vi "EneryPixelInitSingle.vi"(8 "error in (no error)":errorcluster, 11 "MagSpecCamera in":refnum<class "MagSpecCamera.lvclass">) -> (0 "error out":errorcluster, 3 "MagSpecCamera in":refnum<class "MagSpecCamera.lvclass">)   [LabVIEW 2013, in "MagSpecCamera.lvclass"]
uses:
  MagSpecCamera.lvclass
  MagSpecCamera.lvclass/MagSpecCamera.ctl
panel:
  out "Charge Compensation 2":dbl[](graph)
  out "energy dep":dbl[](graph)
  out "Bending angle":dbl[](graph)
  out "Charge Compensation":dbl[](graph)
  out "Momentum [MeV/C]":dbl[](graph)
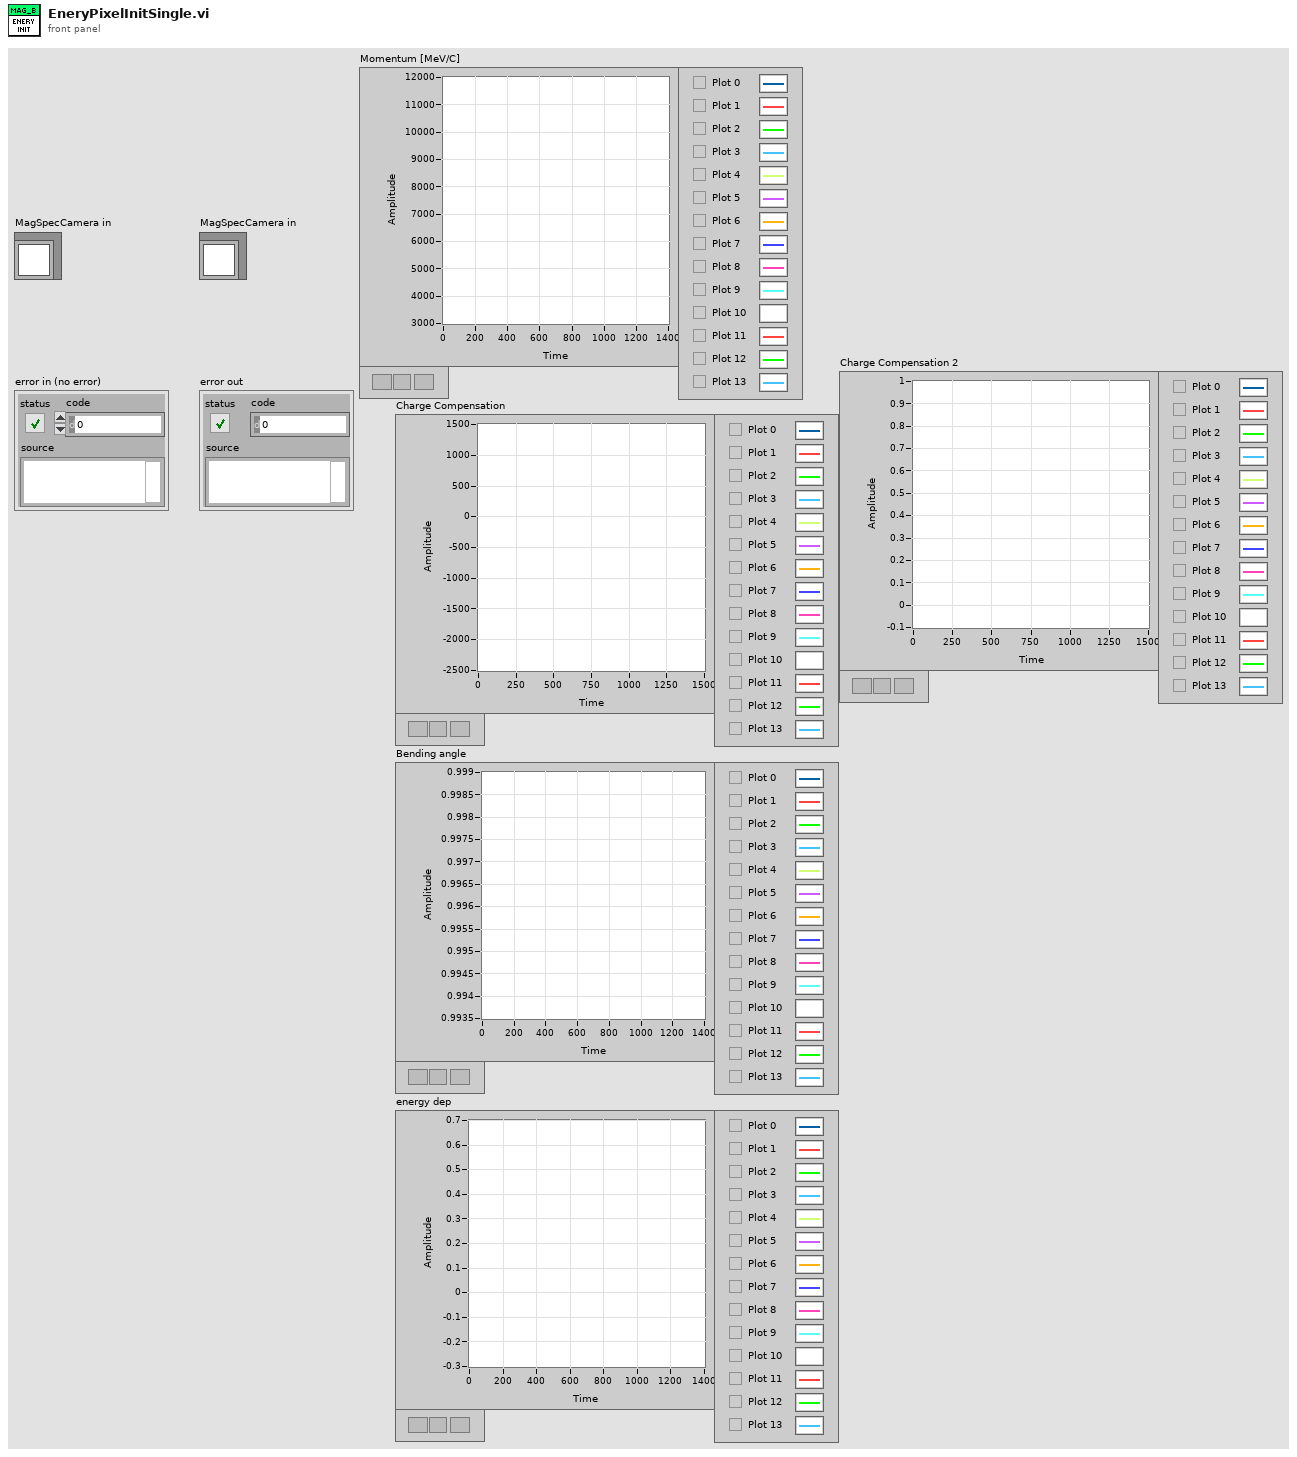
[diagram p1: front panel]
types:
  T1 = typedef "Calibration_Pixel_based.ctl" = cluster{"y1(pixel)":dbl[], "y2(pixel)":dbl[], "dp/B [MeV/C/B] (pixel)":dbl[], "energyDependence Input(pixel)":dbl[], "bending angle [deg](pixel)":dbl[], "total path(pixel)":dbl[], "pixel angle (y)(pixel)":dbl[], "energy dependence (pixel)":dbl[], "charge compensation (pixel)":dbl[], "Momentum [MeV/C](pixel)":dbl[], "angular compensation(pixel)":dbl[]}
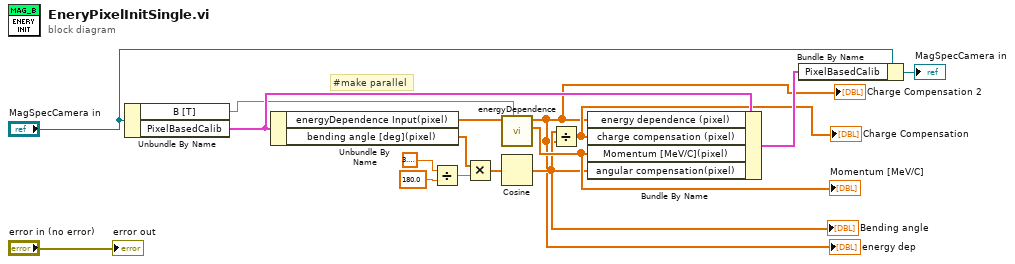
[diagram p0: block diagram]
diagram:
  # "#make parallel"
  n1 = Unbundle By Name("MagSpecCamera in") -> ("B [T]"=w11:dbl, "PixelBasedCalib"=w12:T1)
  n2 = Unbundle By Name(w12) -> ("energyDependence Input(pixel)"=w5:dbl[], "bending angle [deg](pixel)"=w6:dbl[])
  n3 = Divide(x=3.141592653589793, y=180.0) -> (x/y=w2:dbl)
  n4 = Multiply(x=w6, y=w2) -> (x*y=w1:dbl[])
  n5 = call "energyDependence.vi"("B [T]"=w11, "energy vs pixel"=w5) -> ("Momentum [MeV/C] vs pix"=w10:dbl[], "energy dependence"=w7:dbl[])  [unwired: 8 in]
  "Momentum [MeV/C]" <- w10
  "energy dep" <- w7
  "Charge Compensation 2" <- w7
  n6 = Cosine(x=w1) -> (cos(x)=w8:dbl[])
  "Bending angle" <- w8
  n7 = Divide(x=w8, y=w7) -> (x/y=w9:dbl[])
  "Charge Compensation" <- w9
  n8 = Bundle By Name(cluster=w12, "energy dependence (pixel)"=w7, "charge compensation (pixel)"=w9, "Momentum [MeV/C](pixel)"=w10, "angular compensation(pixel)"=w8) -> (w13:T1)
  n9 = Bundle By Name(cluster="MagSpecCamera in", "PixelBasedCalib"=w13) -> (→"MagSpecCamera in":refnum<class "MagSpecCamera.lvclass">)
  "error out" <- "error in (no error)"
